vi "CTRE_PigeonIMU_Open_CAN.vi"(8 "error in":errorcluster, 10 "Device Number":u8) -> (0 "error out":errorcluster, 3 "PigeonIMUDevRef":T1={"DeviceStatus"={"status"=FALSE, "code"=0, "source"=""}, "Device Number"=0, "Type"=352321536, "Device ID"=0} {"Type" items=["CAN"=352321536, "TalonSRX"=33554432]})   [LabVIEW 2016]
uses:
  <vilib>/Rock Robotics/WPI/ThirdParty/Sensors/Pigeon/CTRE_PigeonIMU_DeviceRef.ctl
  <vilib>/Rock Robotics/WPI/ThirdParty/Sensors/Pigeon/CTRE_PigeonIMU_ConnectionType.ctl
  <vilib>/Rock Robotics/WPI/ThirdParty/Sensors/Pigeon/CTRE_PigeonIMU_MessageIDs.ctl
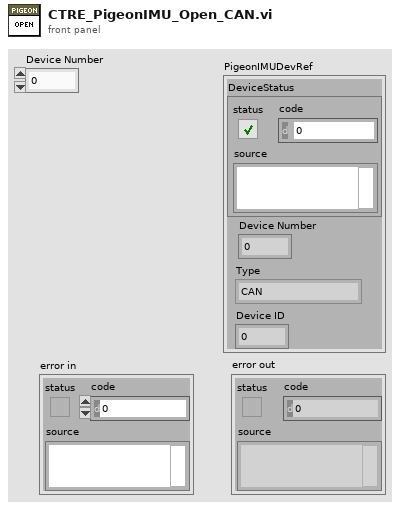
[diagram p1: front panel]
types:
  T1 = typedef "CTRE_PigeonIMU_DeviceRef.ctl" = cluster{"DeviceStatus":errorcluster, "Device Number":u8, "Type":T2, "Device ID":u32}
  T2 = typedef "CTRE_PigeonIMU_ConnectionType.ctl" = u32
  T3 = typedef "CTRE_PigeonIMU_MessageIDs.ctl" = u32
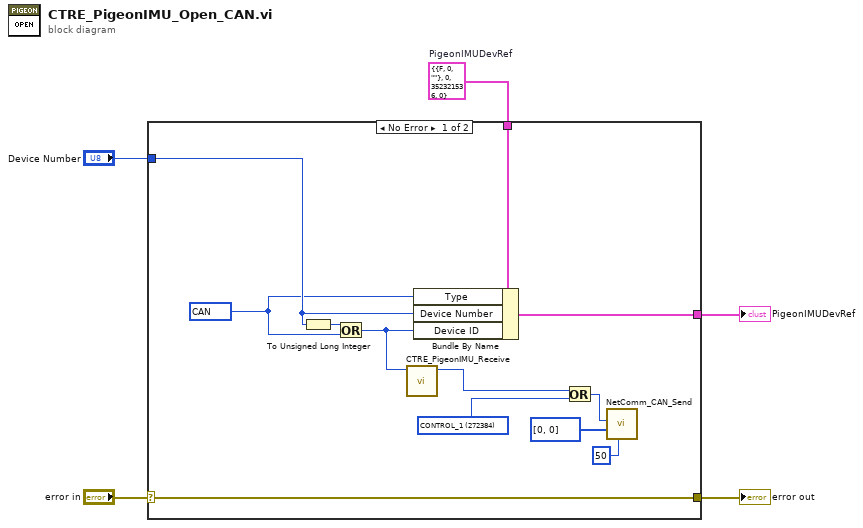
[diagram p0: block diagram]
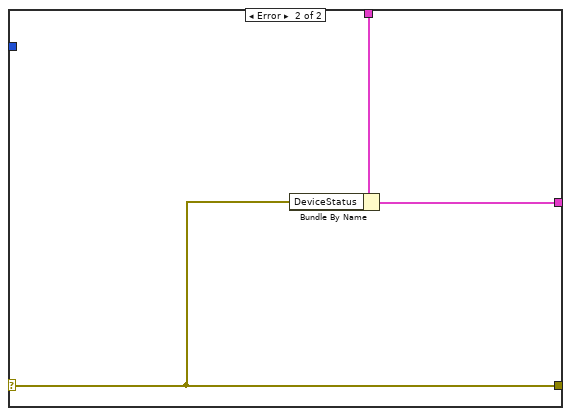
[diagram p2: hidden frame]
diagram:
  w3 = T1 {"DeviceStatus"={"status"=FALSE, "code"=0, "source"=""}, "Device Number"=0, "Type"=352321536, "Device ID"=0}  # PigeonIMUDevRef
  n1 = case shown="No Error" "error in" {
    selector: "error in" -> [w17 w19]
    tunnel: [w17 w19] -> w4
    tunnel: w3 -> [w16 w20]
    tunnel: [w15 w18] -> w2
    tunnel: "Device Number" -> [w13 _]
    frame No Error {
      w6 = T2 352321536 items=["CAN"=352321536, "TalonSRX"=33554432] ("Connection Type")
      w12 = T3 272384 items=["RAW_STATUS_2"=265280, "RAW_STATUS_4"=265408, "RAW_STATUS_6"=265536, "BIASED_STATUS_2"=269376, "BIASED_STATUS_4"=269504, "BIASED_STATUS_6"=269632, "COND_STATUS_1"=270336, "COND_STATUS_2"=270400, "COND_STATUS_3"=270464, "COND_STATUS_4"=270528, "COND_STATUS_5"=270592, "COND_STATUS_6"=270656, "COND_STATUS_7"=270720, "COND_STATUS_8"=270784, "COND_STATUS_9"=270848, "COND_STATUS_10"=270912, "CONTROL_1"=272384, "PARAM_REQUEST"=273408, "PARAM_RESPONSE"=273472, "PARAM_SET"=273536] ("MessageIDs")
      n2 = To Unsigned Long Integer(number=w13) -> (unsigned 32bit integer=w14:u32)
      n3 = Or(x=w14, y=w6) -> (x .or. y?=w8:T2)
      n4 = call <vilib>:"CTRE_PigeonIMU_Receive.vi"("Device ID"=w8) -> ("Device ID Out"=w7:u32)  [unwired: 10 in]
      n5 = Bundle By Name(cluster=w16, "Type"=w6, "Device Number"=w13, "Device ID"=w8) -> (w15:T1)
      n6 = Or(x=w7, y=w12) -> (x .or. y?=w11:T3)
      n7 = call <vilib>:"NetComm_CAN_Send.vi"("Period (ms)"=50, "Data"=u8[] [0, 0], "Message ID"=w11) -> ()  [unwired: 8 in, 1 out]
    }
    frame Error {
      n8 = Bundle By Name(cluster=w20, "DeviceStatus"=w19) -> (w18:T1)
    }
  }
  "error out" <- w4
  "PigeonIMUDevRef" <- w2
